vi "Get_All_Remote_SV_by_IP.vi"(8 "error in (no error)":errorcluster, 9 "timeout (30 s)":i32=30, 11 "IP Address":string="HousesOfTheHoly") -> (0 "error out":errorcluster, 2 "Shared Variable List":refnum<k21>[](array[refnum]), 3 "Processes":T1(array[cluster]))   [LabVIEW 2020]
doc: "This VI gets all the shared variables from a remote target.\n\nCreated By:\nRyan Pacini\n11/31/11"
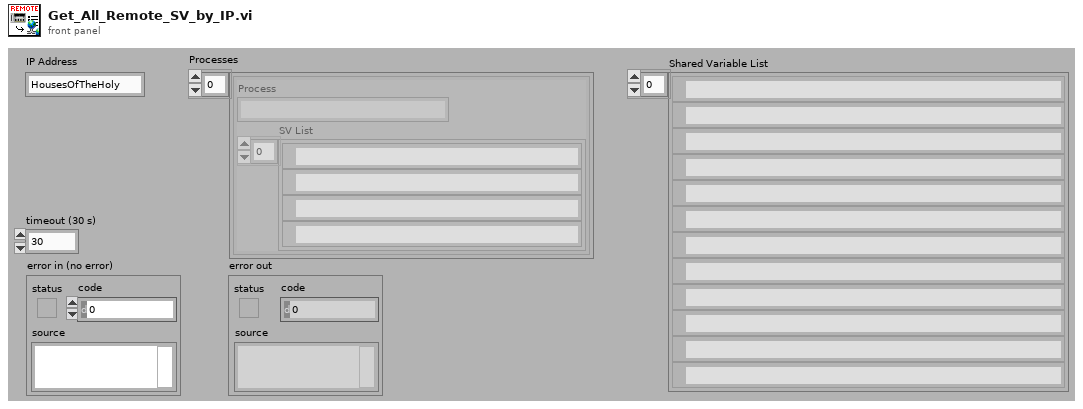
[diagram p1: front panel]
types:
  T1 = cluster{"Process":string, "SV List":refnum<k21>[]}[]
  T2 = cluster{string, "Shared Variable List":refnum<k21>[]}
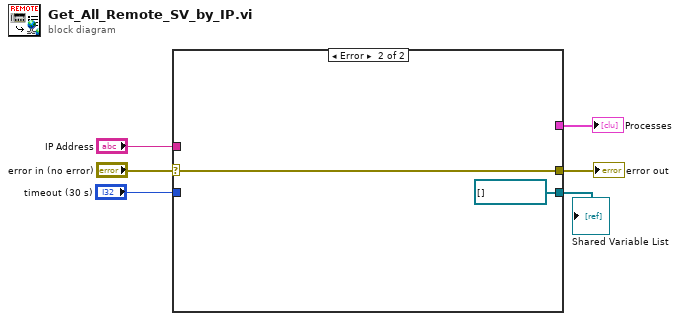
[diagram p0: block diagram]
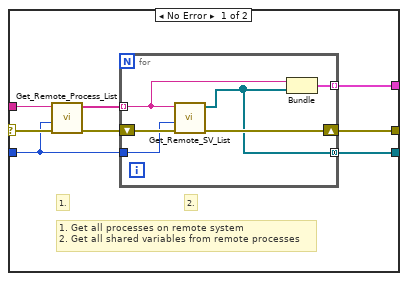
[diagram p2: hidden frame]
diagram:
  n1 = case shown="Error" "error in (no error)" {
    selector: "error in (no error)" -> [w9 w22]
    tunnel: [w12 _] -> w6
    tunnel: "IP Address" -> [w11 _]
    tunnel: [w10 w22] -> w4
    tunnel: "timeout (30 s)" -> [w8 _]
    tunnel: [w7 refnum<k21>[] [] ("Shared Variable List")] -> w1
    frame No Error {
      # "1. Get all processes on remote system\n2. Get all shared variables from remote processes"
      # "2."
      # "1."
      n2 = call "Get_Remote_Process_List.vi"("error in (no error)"=w9, "timeout (30 s)"=w8, "IP Address or PC Name"=w11) -> ("error out"=w14:errorcluster, "Process List (\\\\[IPAddress]\\[Process])"=w13:string[])  [unwired: 7 in]
      n3 = for {
        tunnel: w13 -> [w18] mode=indexing
        shift-right: [w19] -> w10
        shift-left: w14 -> [w20]
        tunnel: [w17] -> w12 mode=indexing
        tunnel: w8 -> [w16]
        tunnel: [w15] -> w7 mode=concatenating
        n4 = call "Get_Remote_SV_List.vi"("error in (no error)"=w20, "timeout (30 s)"=w16, "Process (\\\\[IPAddress]\\[Process])"=w18) -> ("error out"=w19:errorcluster, "Shared Variable List"=w15:refnum<k21>[])  [unwired: 7 in]
        n5 = Bundle(w18, "Shared Variable List"=w15) -> (w17:T2)  [unwired: 1 in]
      }
    }
    frame Error {
    }
  }
  "Processes" <- w6
  "error out" <- w4
  "Shared Variable List" <- w1
